vi "4.4.vi"() -> ()   [LabVIEW 2017]
panel:
  out "强度图":dbl[][](graph)
  out "数组":dbl[][](array[numeric])
  # "任务四"
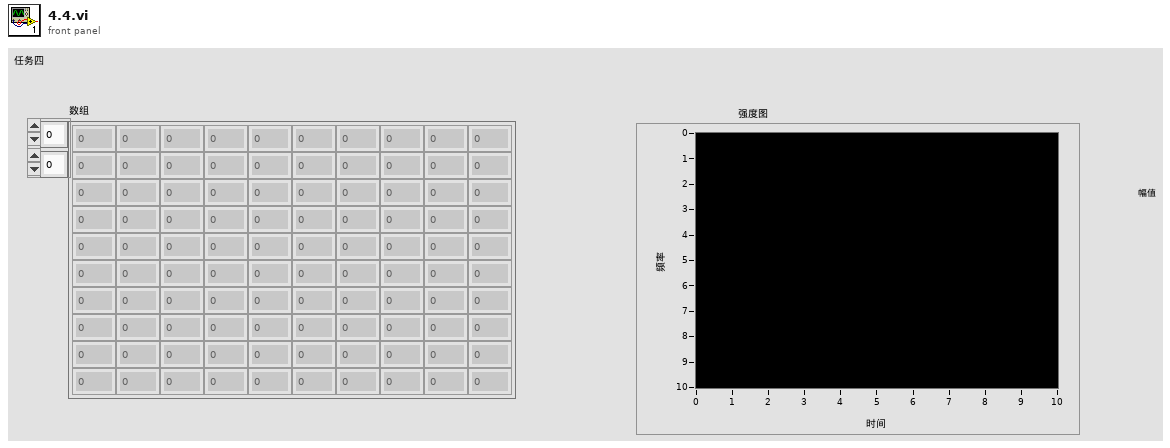
[diagram p1: front panel]
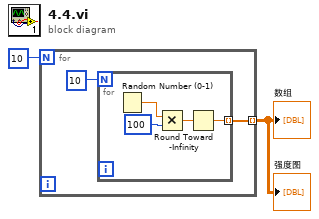
[diagram p0: block diagram]
diagram:
  n1 = for {
    N: 10 -> [_]
    tunnel: [w3] -> w2 mode=indexing
    n2 = for {
      N: 10 -> [_]
      tunnel: [w5] -> w3 mode=indexing
      n3 = Random Number (0-1)() -> (number: 0 to 1=w7:dbl)
      n4 = Multiply(x=w7, y=100) -> (x*y=w6:dbl)
      n5 = Round Toward -Infinity(1:w6) -> (0:w5:dbl)
    }
  }
  "数组" <- w2
  "强度图" <- w2
